vi "Get Test Config File Path.vi"(8 "error in (no error)":errorcluster, 11 "Process Test In":refnum<class "Process Test.lvclass">) -> (0 "error out":errorcluster, 2 "Test config path":path, 3 "Process Test Out":refnum<class "Process Test.lvclass">)   [LabVIEW 2020, in "Process Test.lvclass"]
uses:
  Process Test.lvclass
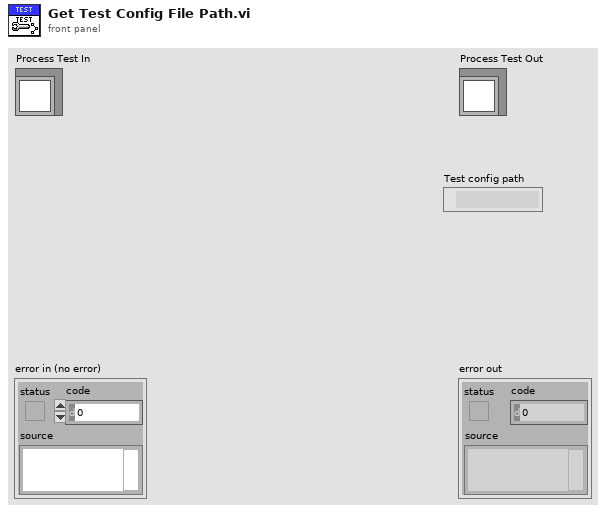
[diagram p1: front panel]
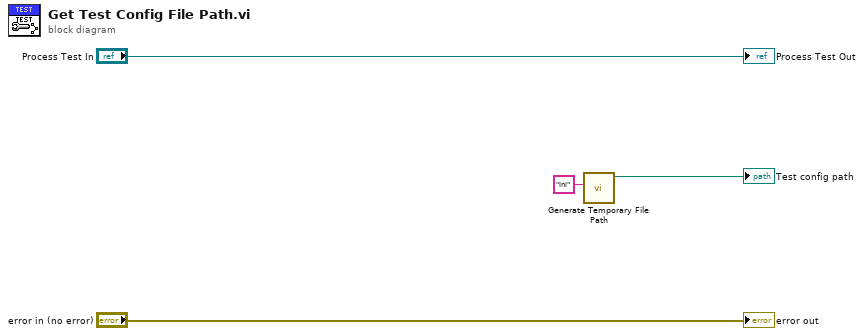
[diagram p0: block diagram]
diagram:
  n1 = call <vilib>:"Generate Temporary File Path.vi"("Temporary File Extension (tmp)"="ini") -> ("Unique Temporary File Path"=→"Test config path":path)  [unwired: 9 in, 1 out]
  "error out" <- "error in (no error)"
  "Process Test Out" <- "Process Test In"
